vi "filter_frequency_imp_test_v4.vi"() -> ()   [LabVIEW 2014]
uses:
  <vilib>/rvi/Analysis/host/Butterworth/config/Butterworth Filter Order.ctl
  <vilib>/rvi/Analysis/host/Butterworth/config/Butterworth Filter Type.ctl
  <vilib>/FPGAPlugInAG/cRIO-9039/niLvFpga_Open_cRIO-9039.vi
  <vilib>/rvi/interface/common/dynamic/niFpgaDynamicAddResources.vi
  <vilib>/rvi/Analysis/host/Butterworth/config/BwScaledCoefficients.vi
  <vilib>/Utility/error.llb/Error Cluster From Error Code.vi
  <vilib>/rvi/errors/niLvFpgaAdjustHostInterfaceError.vi
  <vilib>/FPGAPlugInAG/Dynamic/niLvFpga_Close_Dynamic.vi
  <vilib>/rvi/interface/nirviOpenFPGA/nirviOpenFPGA.xnode
  FPGA Bitfiles/test0304_FPGATarget_imptestv4_skixW0YTJzY.lvbitx
  FPGA VIs/imp_test_v4.vi
  <vilib>/rvi/Analysis/host/Butterworth/XNode/ButterworthCoefficients.xnode
  <vilib>/rvi/interface/nirviReadWriteControl/nirviReadWriteControl.xnode
  <vilib>/rvi/interface/nirviCloseFPGA/nirviCloseFPGA.xnode
  <vilib>/rvi/Analysis/host/Public/NI_FpgaMspHost.lvlib
  NiFpgaLv.dll
  <vilib>/rvi/interface/Simulation/niFpgaSimulationCallBeginRW.vi
panel:
  in  "sr_Strain(Avg.)_p (S/s)":dbl=50000.0
  in  "fcu_Strain(Avg.)_p (Hz)":dbl=1000.0
  in  "sr_Dp_dd (S/s)":dbl=50000.0
  in  "fcu_Dp_dd (Hz)":dbl=1000.0
  in  "sr_dFp_PIS (S/s)":dbl=50000.0
  in  "fcu_dFp_PID (Hz)":dbl=1000.0
  in  "sr_Strain(Avg.)_y (S/s)":dbl=50000.0
  in  "fcu_Strain(Avg.)_y (Hz)":dbl=1000.0
  in  "sr_Dy_dd (S/s)":dbl=50000.0
  in  "fcu_Dy_dd (Hz)":dbl=1000.0
  in  "sr_dFy_PID (S/s)":dbl=50000.0
  in  "fcu_dFy_PID (Hz)":dbl=1000.0
  in  "stop":bool
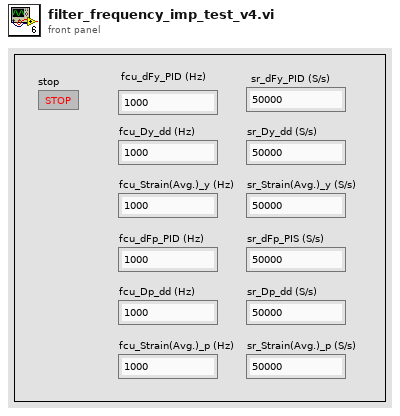
[diagram p1: front panel]
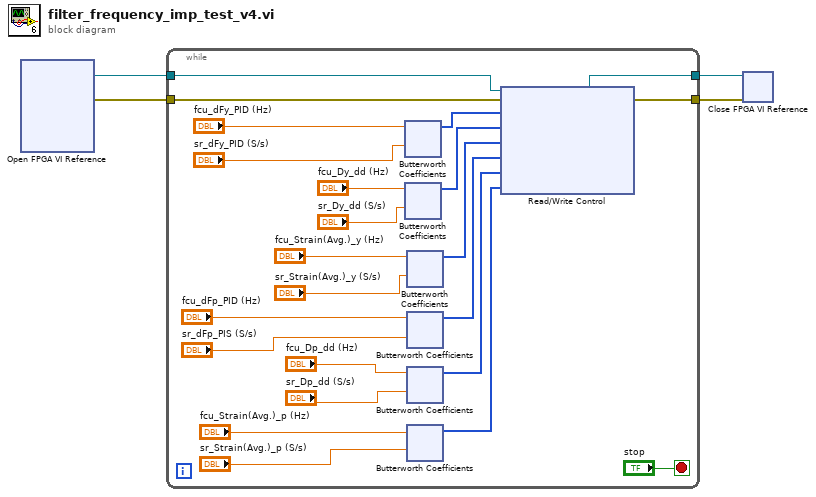
[diagram p0: block diagram]
diagram:
  n1 = xnode "Open FPGA VI Reference"() -> ("FPGA VI Reference Out"=w4:refnum<k20>, "error out"=w3:errorcluster)  [unwired: 2 in]
  n2 = while {
    tunnel: w4 -> [w17]
    tunnel: w3 -> [w26]
    tunnel: [w25] -> w2
    tunnel: [w24] -> w1
    stop <- "stop" stop-if-true
    n3 = xnode "Butterworth Coefficients"("cutoff frequency (Hz)"="fcu_dFy_PID (Hz)", "sample rate (S/s)"="sr_dFy_PID (S/s)") -> ("scaled coefficients"=w16:i32[])  [unwired: 1 in, 1 out]
    n4 = xnode "Butterworth Coefficients"("cutoff frequency (Hz)"="fcu_Dy_dd (Hz)", "sample rate (S/s)"="sr_Dy_dd (S/s)") -> ("scaled coefficients"=w15:i32[])  [unwired: 1 in, 1 out]
    n5 = xnode "Butterworth Coefficients"("cutoff frequency (Hz)"="fcu_Strain(Avg.)_y (Hz)", "sample rate (S/s)"="sr_Strain(Avg.)_y (S/s)") -> ("scaled coefficients"=w14:i32[])  [unwired: 1 in, 1 out]
    n6 = xnode "Butterworth Coefficients"("cutoff frequency (Hz)"="fcu_dFp_PID (Hz)", "sample rate (S/s)"="sr_dFp_PIS (S/s)") -> ("scaled coefficients"=w13:i32[])  [unwired: 1 in, 1 out]
    n7 = xnode "Butterworth Coefficients"("cutoff frequency (Hz)"="fcu_Dp_dd (Hz)", "sample rate (S/s)"="sr_Dp_dd (S/s)") -> ("scaled coefficients"=w12:i32[])  [unwired: 1 in, 1 out]
    n8 = xnode "Butterworth Coefficients"("cutoff frequency (Hz)"="fcu_Strain(Avg.)_p (Hz)", "sample rate (S/s)"="sr_Strain(Avg.)_p (S/s)") -> ("scaled coefficients"=w11:i32[])  [unwired: 1 in, 1 out]
    n9 = xnode "Read/Write Control"("FPGA VI Reference In"=w17, "error in"=w26, "dFy_PID coeff."=w16, "Dy_dd coeff."=w15, "Strain_y mean coeff."=w14, "dFp_PID coeff."=w13, "Dp_dd coeff."=w12, "Strain_p mean coeff."=w11) -> ("FPGA VI Reference Out"=w25:refnum<k20>, "error out"=w24:errorcluster)
  }
  n10 = xnode "Close FPGA VI Reference"("FPGA VI Reference In"=w2, "error in"=w1) -> ()  [unwired: 1 out]
